vi "Abort ROI Creation Global.vi"() -> ()   [LabVIEW 2021, in "Image.lvlib"]
uses:
  Image.lvlib
panel:
  out "Abort ROI Creation":bool
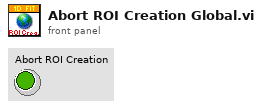
[diagram p1: front panel]
diagram:
